vi "IC_ActiveBuffer_to_IMAQ.vi"(0 "ICImagingControl In":refnum<k7>, 1 "BorderSize":i32=3, 2 "Error In (no error)":errorcluster) -> (3 "ICImagingControl Out":refnum<k7>, 4 "Image Out":T1, 5 "SampleStartTime":dbl, 6 "Error Out":errorcluster)   [LabVIEW 2020]
uses:
  <vilib>/vision/Image Controls.llb/IMAQ Image.ctl
  IC LabVIEW Extension 2.dll
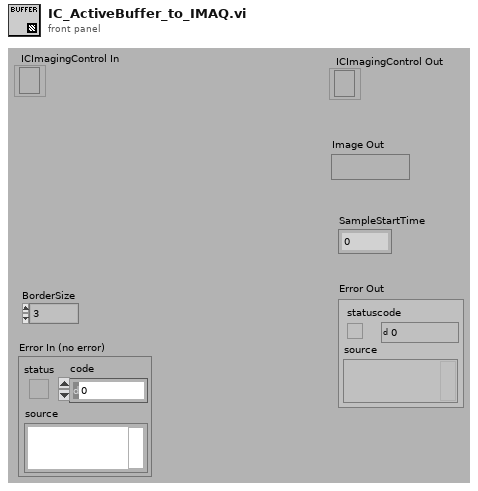
[diagram p1: front panel]
types:
  T1 = typedef "IMAQ Image.ctl" = refnum<image>
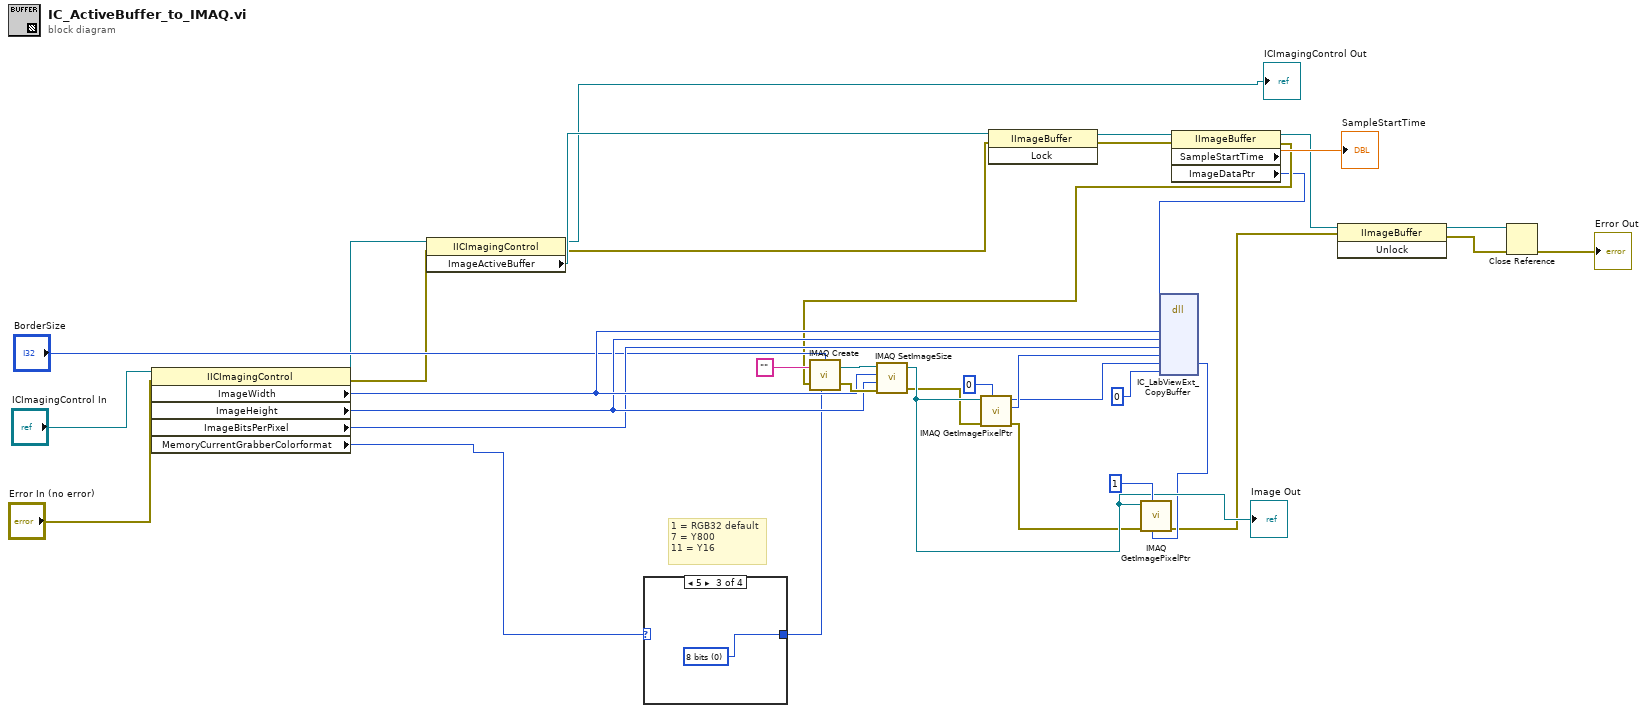
[diagram p0: block diagram]
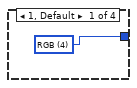
[diagram p2: hidden frame]
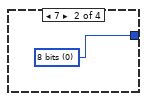
[diagram p3: hidden frame]
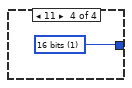
[diagram p4: hidden frame]
diagram:
  # "1 = RGB32 default\n7 = Y800\n11 = Y16"
  n1 = property class="IICImagingControl"(reference="ICImagingControl In", error in="Error In (no error)") -> (reference out=w5:refnum<k7>, error out=w1:errorcluster, "ImageWidth"=w27:i32, "ImageHeight"=w26:i32, "ImageBitsPerPixel"=w25:i32, "MemoryCurrentGrabberColorformat"=w7:i32)
  n2 = property class="IICImagingControl"(reference=w5, error in=w1) -> (reference out=→"ICImagingControl Out":refnum<k7>, error out=w2:errorcluster, "ImageActiveBuffer"=w4:refnum<k7>)
  n3 = case shown="5" w7 {
    tunnel: [w36 w37 w38 w39] -> w6
    frame 1, Default {
      w36 = u32 4 items=["8 bits", "16 bits", "Float", "Complex", "RGB", "HSL"] ("Image Type")
    }
    frame 7 {
      w37 = u32 0 items=["8 bits", "16 bits", "Float", "Complex", "RGB", "HSL"] ("Image Type")
    }
    frame 5 {
      w38 = u32 0 items=["8 bits", "16 bits", "Float", "Complex", "RGB", "HSL"] ("Image Type")
    }
    frame 11 {
      w39 = u32 1 items=["8 bits", "16 bits", "Float", "Complex", "RGB", "HSL"] ("Image Type")
    }
  }
  n4 = invoke class="IImageBuffer" method="Lock"(reference=w4, error in=w2) -> (reference out=w8:refnum<k7>, error out=w9:errorcluster)  [unwired: 1 in, 1 out]
  n5 = property class="IImageBuffer"(reference=w8, error in=w9) -> (reference out=w11:refnum<k7>, error out=w12:errorcluster, "SampleStartTime"=→"SampleStartTime":dbl, "ImageDataPtr"=w10:i32)
  n6 = call "IMAQ Create"("Border Size"="BorderSize", "Image Name"="", "Image Type"=w6, "error in (no error)"=w12) -> ("New Image"=w34:T1, "error out"=w31:errorcluster)  [unwired: 1 in]
  n7 = call "IMAQ SetImageSize"("error in (no error)"=w31, "Y Resolution"=w26, "X Resolution"=w27, "Image"=w34) -> ("error out"=w30:errorcluster, "Image Out"=w32:T1)  [unwired: 1 in]
  "Image Out" <- w32
  n8 = call "IMAQ GetImagePixelPtr"("Function"=0, "error in (no error)"=w30, "Image"=w32) -> ("error out"=w29:errorcluster, "LineWidth(Pixels)"=w24:i32, "Pixel Pointer out"=w23:u64)  [unwired: 3 in, 3 out]
  n9 = dll-call lib="C:/data/documents/Fritz-Haber-Institut/Github/ARPEScontrol/subvi/IC/IC LabVIEW Extension 2.dll" fn="IC_LabViewExt_CopyBuffer"("data"=w10, "width"=w27, "height"=w26, "bpp"=w25, "imaq_width"=w24, "imaq_ptr"=w23, "bFlip"=0) -> ("imaq_ptr"=w21:u32)  [unwired: 10 in, 2 out]
  n10 = call "IMAQ GetImagePixelPtr"("Pixel Pointer in"=w21, "Function"=1, "error in (no error)"=w29, "Image"=w32) -> ("error out"=w16:errorcluster)  [unwired: 2 in, 5 out]
  n11 = invoke class="IImageBuffer" method="Unlock"(reference=w11, error in=w16) -> (reference out=w15:refnum<k7>, error out=w14:errorcluster)  [unwired: 1 in, 1 out]
  n12 = Close Reference(reference=w15, error in (no error)=w14) -> (error out=→"Error Out":errorcluster)
